vi "Wave Generation.vi"(2 "Pixel time (tick)":i32=80, 3 "Num of elements":u32=512000, 5 "Elements per line":i32=1000, 6 "Num of undershoot":i32=50, 7 "Resolution":i32=512, 8 "Pixel pulse_initial delay":i32=1, 9 "Pixel clock_pulse width(tick)":i32=40, 10 "Frame retrace time":u32=100 caption="Frame retrace time (ms)") -> (12 "Frame waveform output finish?":bool, 13 "Line clock":bool, 16 "Request address":u32, 17 "Galvo signal readed":u32, 18 "Data":u32, 19 "Pixel clock":bool)   [LabVIEW 2015]
uses:
  <vilib>/Platform/TimedLoop/XDataNode/wakeup.ctl
  <vilib>/Platform/TimedLoop/XDataNode/XDNodeRunTimeDep.lvlib
  <vilib>/Platform/TimedLoop/XDataNode/nitl_modes.ctl
  <vilib>/Platform/TimedLoop/XDataNode/timing_clust.ctl
  <vilib>/Platform/TimedLoop/XDataNode/XDataNode.xnode
  <vilib>/eio/EIONode/EIONode.xnode
  <vilib>/rvi/eio/common/nirviEmuTemplateMethod_errors.vi
  Globals/Global_Sample per Frame.vi
  OpenScan Labview code_20170126/DRAM data index.ctl
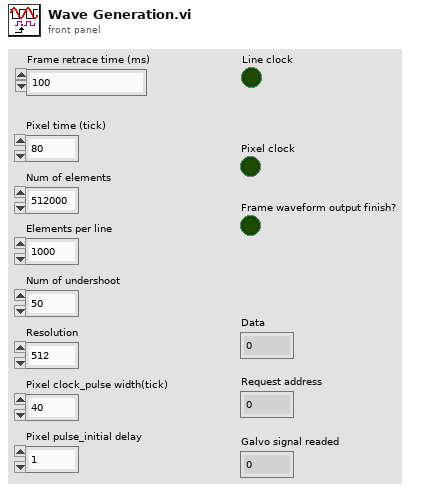
[diagram p1: front panel]
types:
  T1 = typedef "XDNodeRunTimeDep.lvlib/timing_clust.ctl" = cluster{"Expected End [f-1]":u64, "Actual End [f-1]":u64, "Finished Late? [f-1]":bool, "Expected End [i-1]":u64, "Actual End [i-1]":u64, "Finished Late? [i-1]":bool, "Expected Start [i]":u64, "Actual Start [i]":u64, "Expected Start [f]":u64, "Actual Start [f]":u64, "Source Name":string, "Structure Name":string, "Period":i64, "Deadline":i64, "Offset":i64, "Start":i64, "Priority":i32, "Timeout":i32, "Mode":T2, "Wakeup Reason":T3, "Error":errorcluster, "Source Type":string, "Secondary Source Type":string, "Global End Time":u64, "Global Start Time":u64, "Frame Duration":u64, "Iteration Duration":u64, "Assigned CPU":i32, "I/O Scan Engine Mode":u32}
  T2 = typedef "XDNodeRunTimeDep.lvlib/nitl_modes.ctl" = enum32{"No Change", "Process missed periods, maintain original phase", "Discard missed periods, maintain original phase", "Process missed periods, ignore original phase", "Discard missed periods, ignore original phase"}
  T3 = typedef "XDNodeRunTimeDep.lvlib/wakeup.ctl" = enum32{"Normal", "Aborted", "Asynchronous wakeup", "Timing source error", "Timed loop error", "Timeout"}
  T4 = typedef "DRAM data index.ctl" = enum16{"Numeric 1", "Numeric 2", "Numeric 3", "Numeric 4", "Numeric 5", "Numeric 6", "Numeric 7", "Numeric 8", "Numeric 9", "Numeric 10", "Numeric 11", "Numeric 12", "Numeric 13", "Numeric 14", "Numeric 15", "Numeric 16"}
  T5 = cluster{"Numeric 1":u32, "Numeric 2":u32, "Numeric 3":u32, "Numeric 4":u32, "Numeric 5":u32, "Numeric 6":u32, "Numeric 7":u32, "Numeric 8":u32, "Numeric 9":u32, "Numeric 10":u32, "Numeric 11":u32, "Numeric 12":u32, "Numeric 13":u32, "Numeric 14":u32, "Numeric 15":u32, "Numeric 16":u32}
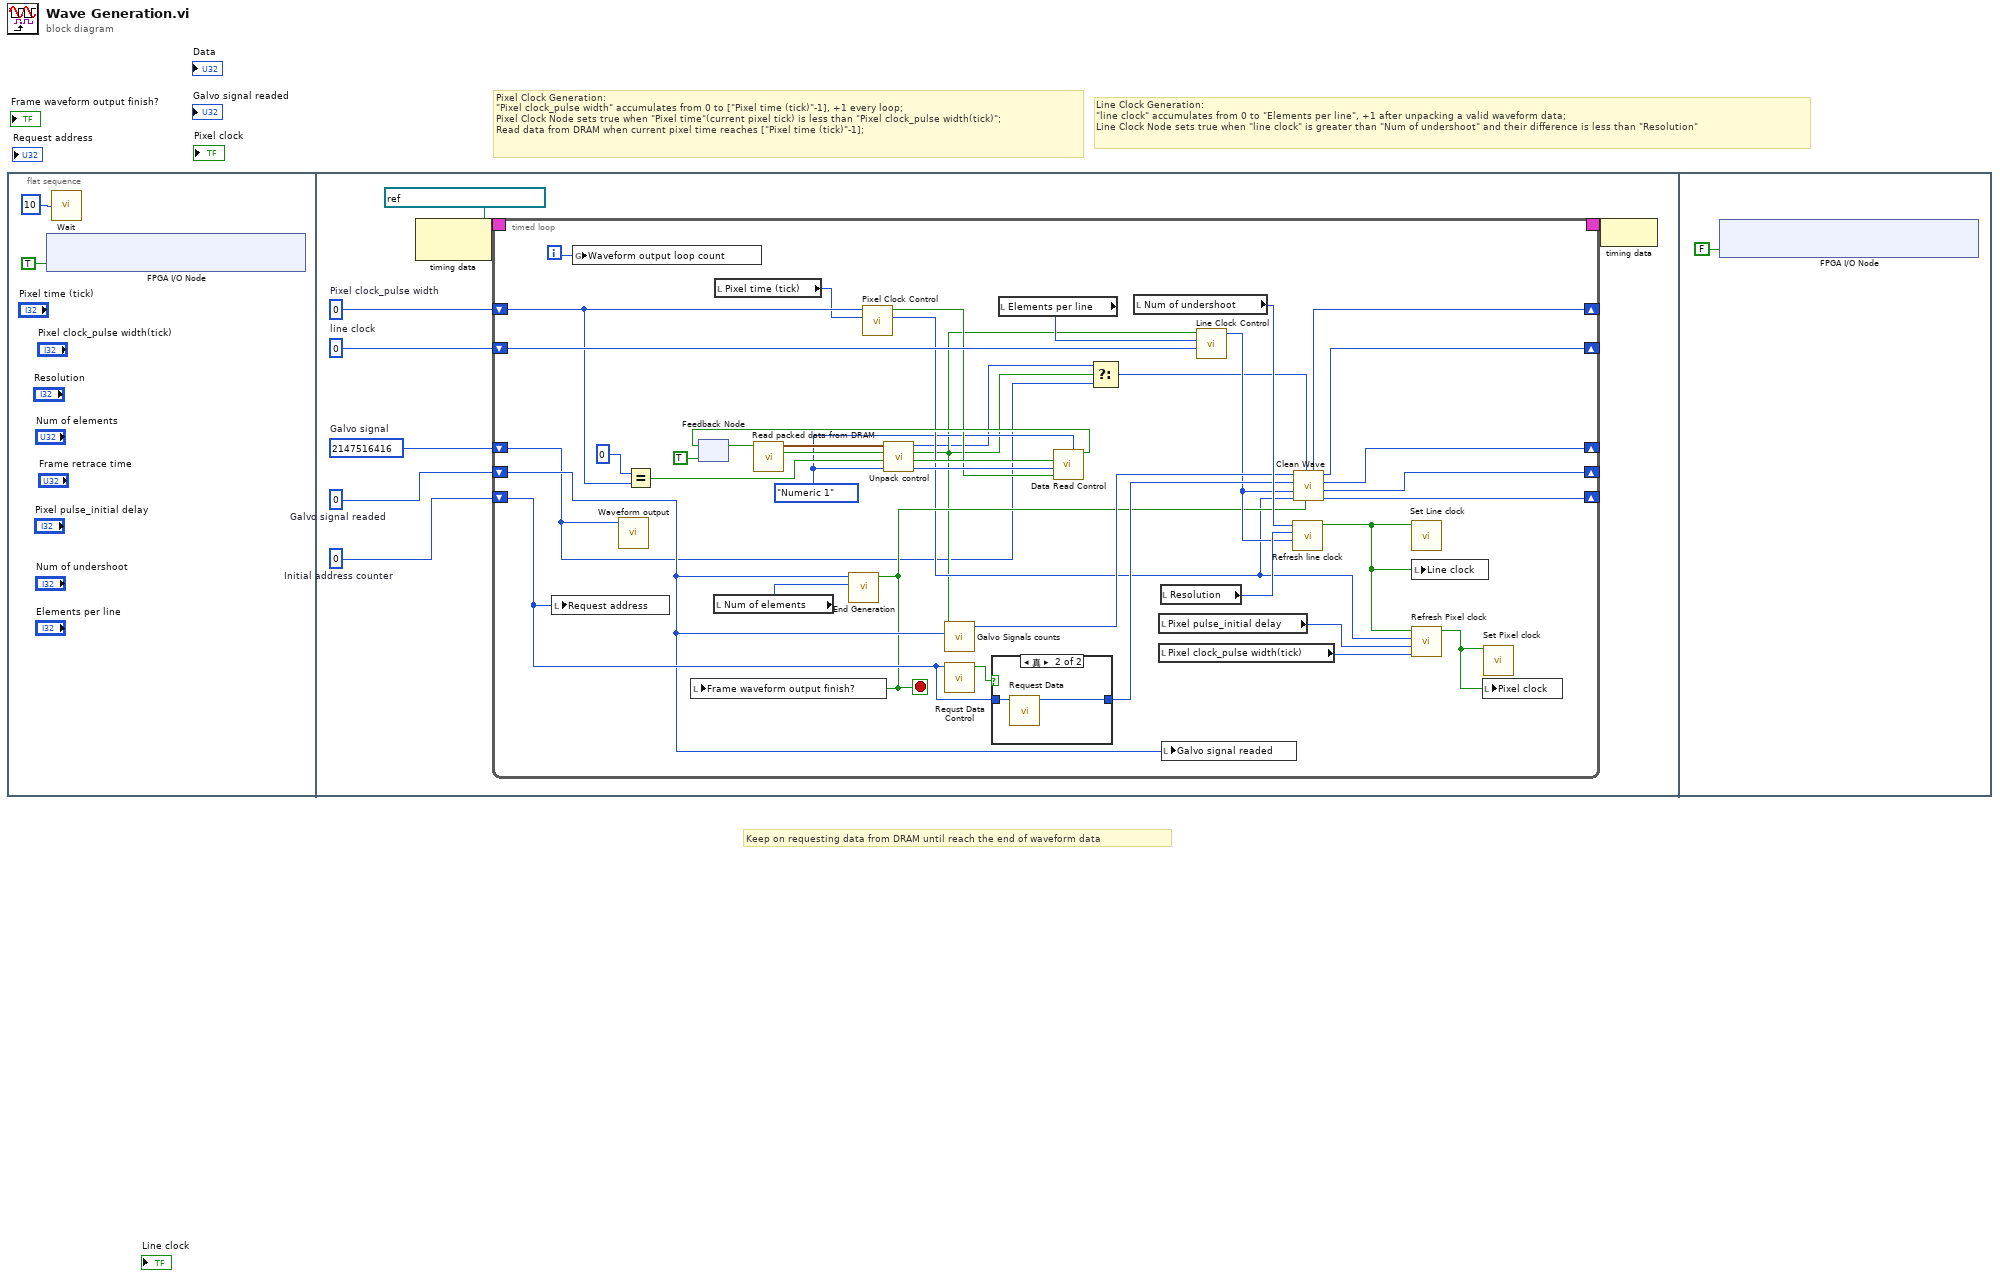
[diagram p0: block diagram]
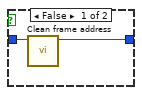
[diagram p2: hidden frame]
diagram:
  # "Keep on requesting data from DRAM until reach the end of waveform data"
  # "Line Clock Generation:\n\"line clock\" accumulates from 0 to \"Elements per line\", +1 after unpacking a valid waveform data;\nLine Clock Node sets true when \"line clock\" is greater than \"Num of undershoot\" and their difference is less than \"Resolution\""
  # "Pixel Clock Generation: \n\"Pixel clock_pulse width\" accumulates from 0 to [\"Pixel time (tick)\"-1], +1 every loop;\nPixel Clock Node sets true when \"Pixel time\"(current pixel tick) is less than \"Pixel clock_pulse width(tick)\";\nRead data from DRAM when current pixel time reaches [\"Pixel time (tick)\"-1];"
  n1 = flat-sequence {
    frame #0 {
      n2 = xnode "FPGA I/O Node"("IO Module\\Shutter(DDCA_PFI1_WRITE)"=TRUE ("IO Module\\Shutter(DDCA_PFI1_WRITE)")) -> ()  [unwired: 1 in, 1 out]
      n3 = call "Wait"("Count(uSec)"=u32 10) -> ()  [unwired: 1 out]
    }
    frame #1 {
      w7 = u32 0  # Initial address counter
      w3 = 0  # Pixel clock_pulse width
      w4 = 0  # line clock
      w5 = u32 0  # Galvo signal readed
      w6 = u32 2147516416  # Galvo signal
      n4 = node-c288(refnum<k21> "40 MHz Onboard Clock" ("Source Name")) -> (w10:T1)
      n5 = timed-loop {
        timing: w10 -> [_]
        timing-out: [_] -> w9
        shift-right: [w20] -> _
        shift-left: w7 -> [w49]
        shift-right: [w23] -> _
        shift-left: w6 -> [w14]
        shift-right: [w22] -> _
        shift-left: w5 -> [w47]
        shift-right: [w21] -> _
        shift-left: w4 -> [w50]
        shift-right: [w11] -> _
        shift-left: w3 -> [w48]
        i -> [w33]
        stop <- w19 stop-if-true
        w16 = DRAM_data_index."Numeric 1" ("DRAM pack index out")
        n6 = local write "Request address"(w49) -> ()
        n7 = global write "Global_Sample per Frame.vi" "Waveform output loop count"(w33) -> ()
        n8 = call "Waveform output.vi"("Galvo signal"=w14) -> ()  [unwired: 11 in]
        n9 = Equal?(x=0, y=w48) -> (x = y?=w39:bool)
        n10 = feedback #1(TRUE) -> (w41:bool)
        n11 = local read "Num of elements"() -> (w34:u32)
        n12 = local read "Pixel time (tick)"() -> (w38:i32)
        n13 = call "Read packed data from DRAM.vi"("Output ready"=w41) -> ("Output Valid§"=w45:bool, "Data"=w44:T5)  [unwired: 9 in]
        n14 = call "End Generation.vi"("Num of elements"=w34, "Galvo signal readed"=w47) -> ("End Generation"=w19:bool)  [unwired: 9 in]
        n15 = local write "Frame waveform output finish?"(w19) -> ()
        n16 = call "Pixel Clock Control.vi"("Pixel time (tick)"=w38, "Pixel clock_pulse width"=w48) -> ("Pixel time"=w18:i32, "Pixel time up"=w17:bool)  [unwired: 8 in]
        n17 = call "Unpack control.vi"("DRAM pack index init"=w16, "enable unpack"=w39, "input valid"=w45, "Data"=w44) -> ("output valid?"=w37:bool, "output valid? 2"=w15:bool, "Unpacked data"=w13:u32, "DRAM pack index out out"=w35:T4)  [unwired: 4 in]
        n18 = call "Galvo Signals counts.vi"("Galvo signal readed in"=w47, "output valid? in"=w15) -> ("Galvo signal readed out"=w26:u32)  [unwired: 9 in]
        n19 = call "Requst Data Control.vi"("Initial address counter"=w49) -> ("Enable request"=w42:bool)  [unwired: 10 in]
        n20 = case shown="真" w42 {
          tunnel: w49 -> [w51 w54]
          tunnel: [w52 w53] -> w25
          frame False {
            n21 = call "Clean frame address.vi"("Initial address counter in"=w51) -> ("Initial address counter out"=w52:u32)  [unwired: 10 in]
          }
          frame True {
            n22 = call "Request Data.vi"("Address counter"=w54) -> ("Address counter output"=w53:u32)  [unwired: 10 in]
          }
        }
        n23 = local read "Elements per line"() -> (w46:i32)
        n24 = call "Data Read Control.vi"("DRAM pack index out"=w16, "Pixel time up"=w17, "DRAM pack index out out"=w35, "input valid?"=w37) -> ("output valid"=w36:bool)  [unwired: 7 in]
        n25 = feedback-in #1(w36) -> ()
        n26 = Select(t=w13, s=w15, f=w14) -> (s? t:f=w12:u32)
        n27 = local read "Num of undershoot"() -> (w31:i32)
        n28 = local read "Pixel pulse_initial delay"() -> (w29:i32)
        n29 = local read "Pixel clock_pulse width(tick)"() -> (w28:i32)
        n30 = local read "Resolution"() -> (w32:i32)
        n31 = local write "Galvo signal readed"(w47) -> ()
        n32 = call "Line Clock Control.vi"("line clock in"=w50, "Elements per line"=w46, "output valid? in"=w15) -> ("line clock out"=w24:i32)  [unwired: 8 in]
        n33 = call "Refresh line clock.vi"("line clock output"=w24, "Resolution"=w32, "Num of undershoot"=w31) -> ("Refresh?"=w30:bool)  [unwired: 8 in]
        n34 = call "Clean Wave.vi"("line clock out"=w24, "Galvo signal in"=w12, "pixel clock_pulse width in"=w18, "Clean wave"=w19, "Address counter output"=w25, "Galvo signal readed out"=w26) -> ("Address counter"=w20:u32, "Galvo signal readed out"=w22:u32, "Galvo signal in"=w23:u32, "line clock"=w21:i32, "pixel clock_pulse width out"=w11:i32)  [unwired: 1 in]
        n35 = call "Set Line clock.vi"("Refresh"=w30) -> ()  [unwired: 11 in]
        n36 = local write "Line clock"(w30) -> ()
        n37 = call "Refresh Pixel clock.vi"("Pixel clock_pulse width(tick)"=w28, "Pixel pulse_initial delay"=w29, "Pixel clock_pulse width"=w18, "Refresh input"=w30) -> ("Refresh output"=w27:bool)  [unwired: 7 in]
        n38 = local write "Pixel clock"(w27) -> ()
        n39 = call "Set Pixel clock.vi"("Refresh"=w27) -> ()  [unwired: 11 in]
      }
      n40 = node-c288(w9) -> ()
    }
    frame #2 {
      n41 = xnode "FPGA I/O Node"("IO Module\\Shutter(DDCA_PFI1_WRITE)"=FALSE ("IO Module\\Shutter(DDCA_PFI1_WRITE)")) -> ()  [unwired: 1 in, 1 out]
    }
  }
